vi "Connection_Management_Unit_Test.vi"() -> ()   [LabVIEW 2017]
uses:
  Controls/Packet/Packet.ctl
  Controls/Packet/Packet_Direction.ctl
  Controls/Packet/Packet_Type.ctl
  Controls/Packet/Packet_Priority.ctl
  Controls/Control Packets/CM_Param.ctl
  Controls/Connection Management/Connection_Management_Commands.ctl
panel:
  in  "Commands":T1
  out "Network Error Status":T2(ring)
  in  "Timeout (ms)":i32
  in  "Number of tries":u8
  out "CM Params Out":T3
  out "CM Packet Out":T4
  in  "CM Packet In":T4
  in  "baud rate":u32=9600
  in  "COM Port In":refnum<visa-resource-name>
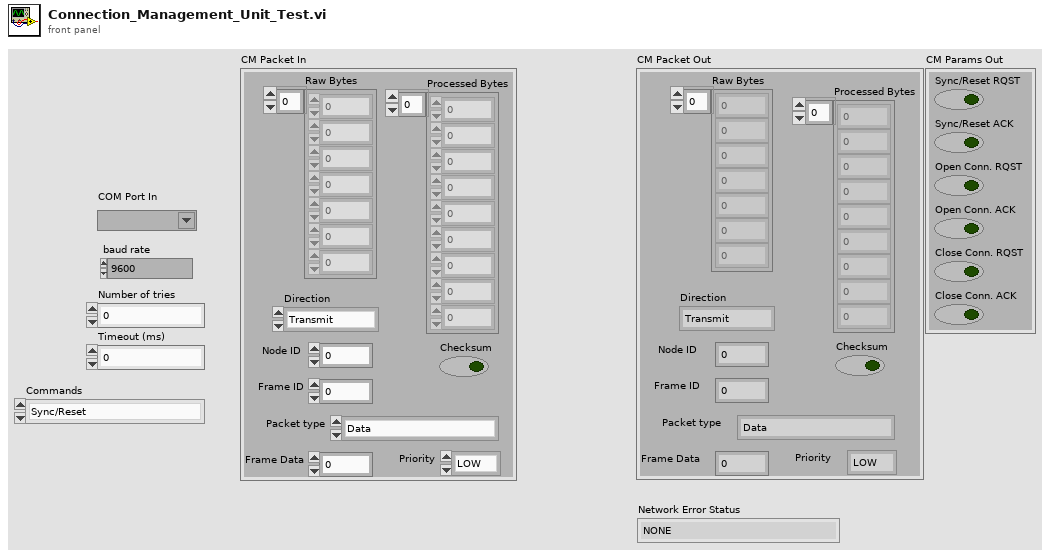
[diagram p1: front panel]
types:
  T1 = typedef "Connection_Management_Commands.ctl" = enum16{"Sync/Reset", "Open Connection", "Close Connection"}
  T2 = enum16{"NONE", "CONNECTION_ALREADY_OPEN", "CONNECTION_ALREADY_CLOSED", "INVALID_FRAME_REQUEST"}
  T3 = typedef "CM_Param.ctl" = cluster{"Sync/Reset RQST":bool, "Sync/Reset ACK":bool, "Open Conn. RQST":bool, "Open Conn. ACK":bool, "Close Conn. RQST":bool, "Close Conn. ACK":bool}
  T4 = typedef "Packet.ctl" = cluster{"Raw Bytes":u8[], "Checksum":bool, "Direction":T5, "Processed Bytes":u8[], "Node ID":u8, "Packet type":T6, "Frame Data":u32, "Priority":T7, "Frame ID":u8}
  T5 = typedef "Packet_Direction.ctl" = enum16{"Transmit", "Receive", "Bidirectional"}
  T6 = typedef "Packet_Type.ctl" = enum16{"Data", "Connection Management", "Remote Request", "Error/Status"}
  T7 = typedef "Packet_Priority.ctl" = enum16{"LOW", "HIGH"}
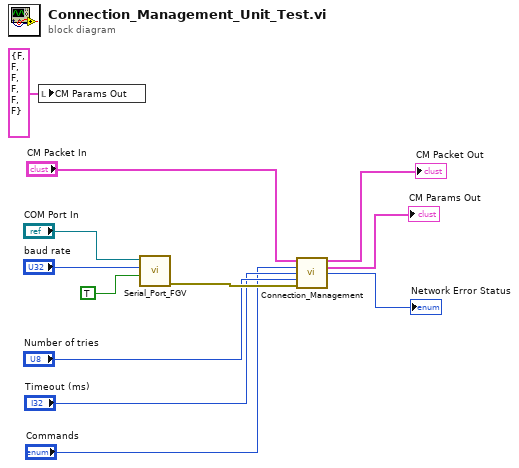
[diagram p0: block diagram]
diagram:
  n1 = local write "CM Params Out"(T3 {"Sync/Reset RQST"=FALSE, "Sync/Reset ACK"=FALSE, "Open Conn. RQST"=FALSE, "Open Conn. ACK"=FALSE, "Close Conn. RQST"=FALSE, "Close Conn. ACK"=FALSE} ("CM Params Out")) -> ()
  n2 = call "Serial_Port_FGV.vi"("Initialize ?"=TRUE, "baud rate"="baud rate", "COM Port In"="COM Port In") -> ("error out"=w9:errorcluster)  [unwired: 7 in, 1 out]
  n3 = call "Connection_Management.vi"("CM Packet In"="CM Packet In", "Commands"="Commands", "Retry interval (ms)"="Timeout (ms)", "Number of tries"="Number of tries", "error in (no error)"=w9) -> ("CM Packet Out"=→"CM Packet Out":T4, "CM Params Out"=→"CM Params Out":T3, "Network Error Status"=→"Network Error Status":T2)  [unwired: 7 in, 1 out]
